vi "Get All Keys.vi"(8 "error in (no error)":errorcluster, 11 "Configuration In":refnum<class "Mock Configuration.lvclass">) -> (0 "error out":errorcluster, 1 "Keys":string[](array[string]), 3 "Configuration Out":refnum<class "Mock Configuration.lvclass">)   [LabVIEW 2020, in "Mock Configuration.lvclass"]
doc: "High-level function for reading configuration file data from process class."
uses:
  Mock Configuration.lvclass
  C:/Program Files (x86)/National Instruments/LabVIEW 2020/vi.lib/Astemes/LMock/Mock.lvclass
  <vilib>/Astemes/LMock/Mock.lvclass
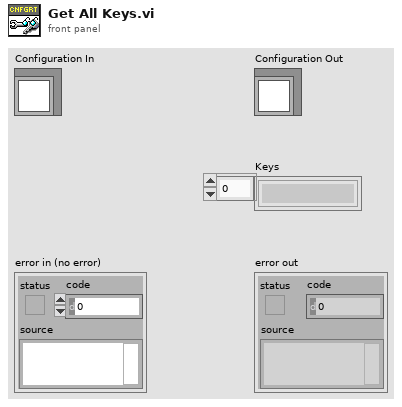
[diagram p1: front panel]
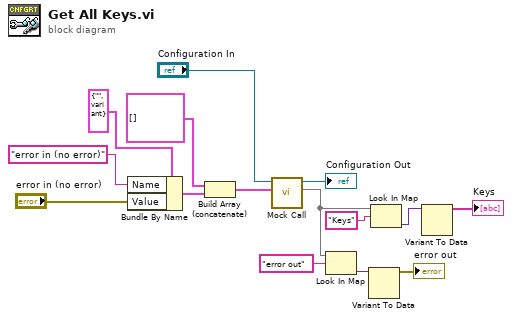
[diagram p0: block diagram]
diagram:
  n1 = Bundle By Name(cluster=cluster{"Name":string, "Value":variant} {"Name"="", "Value"=variant} ("element"), "Name"="error in (no error)", "Value"="error in (no error)") -> (w1:cluster{"Name":string, "Value":variant})
  n2 = Build Array (concatenate)(cluster{"Name":string, "Value":variant}[] [] ("Control Values"), w1) -> (w12:cluster{"Name":string, "Value":variant}[])
  n3 = call <vilib>:"Mock Call.vi"("Control Values"=w12, "Mock In"="Configuration In") -> ("Return Values"=w10:map{string, variant}, "Mock Out"=→"Configuration Out":refnum<class "Mock Configuration.lvclass">)  [unwired: 8 in]
  n4 = Look In Map(map=w10, key="error out") -> (value=w5:variant)  [unwired: 1 in, 1 out]
  n5 = Variant To Data(Variant=w5) -> (data=→"error out":errorcluster)  [unwired: 2 in, 1 out]
  n6 = Look In Map(map=w10, key="Keys") -> (value=w8:variant)  [unwired: 1 in, 1 out]
  n7 = Variant To Data(Variant=w8) -> (data=→"Keys":string[])  [unwired: 2 in, 1 out]
